vi "Save PNG Screenshot.vi"(1 "image data":T1, 5 "Error In":errorcluster) -> (12 "Path":path, 19 "Error Out":errorcluster)   [LabVIEW 2015]
uses:
  <vilib>/picture/picture.llb/imagedata.ctl
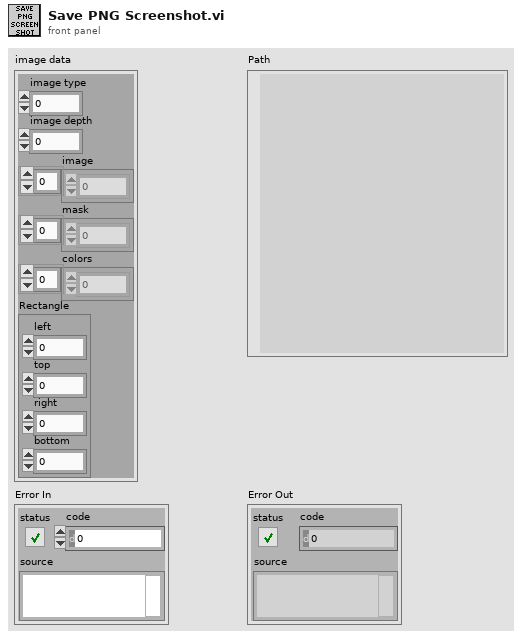
[diagram p1: front panel]
types:
  T1 = typedef "imagedata.ctl" = cluster{"image type":i32, "image depth":i32, "image":u8[], "mask":u8[], "colors":u32[], "Rectangle":cluster{"left":i16, "top":i16, "right":i16, "bottom":i16}}
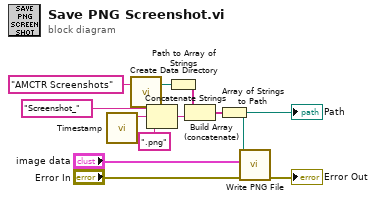
[diagram p0: block diagram]
diagram:
  n1 = call "Timestamp.vi"() -> ("Timestamp String"=w5:string)  [unwired: 11 in]
  n2 = call "Create Data Directory.vi"("Folder Name"="AMCTR Screenshots" ("element")) -> ("Path"=w11:path)  [unwired: 2 in]
  n3 = Concatenate Strings("Screenshot_" ("string"), w5, ".png") -> (w9:string)
  n4 = Path to Array of Strings(0:w11) -> (2:w7:string[])  [unwired: 1 out]
  n5 = Build Array (concatenate)(w7, w9) -> (w10:string[])
  n6 = Array of Strings to Path(0:w10) -> (2:w4:path)  [unwired: 1 in]
  "Path" <- w4
  n7 = call <vilib>:"Write PNG File.vi"("error in (no error)"="Error In", "image data"="image data", "path to PNG file"=w4) -> ("error out"=→"Error Out":errorcluster)  [unwired: 7 in, 1 out]
